vi "Initialize Source.vi"(0 "Intrument Handle[]":refnum<k15>[](array[refnum]), 2 "Channel Number":string[](array[string]), 5 "Measurement Configuration":T1={"Quick Power Down"=FALSE, "Pin Name"=[], "Source Mode"=[], "Start Value"=[], "Target Value"=[], "Compliance Limit"=[], "Sense Mode"=[], "Default Ramp Rate"=[], "Ramp Rate"=[], "Start Delay"=[], "Relative To"=[], "Transient Response"=[], "Data Capture"=FALSE, "Power line frequency"=1} {"Power line frequency" items=["50 Hz", "60 Hz"]; "Start Value" format="%#_6p"; "Transient Response" items=["Slow", "Normal", "Fast"]; "Sense Mode" items=["Local Sense", "Remote Sense"]; "Relative To" items=["Power sequence start", "Previous source start", "Previous source end"]; "Target Value" format="%#_6p"; "Source Mode" items=["DC Voltage", "DC Current"]; "Start Delay" format="%#_6p"; "Compliance Limit" format="%#_6p"; "Ramp Rate" format="%#_6p"}, 11 "error in (no error)":errorcluster) -> (4 "Intrument Handle out[]":refnum<k15>[](array[refnum]), 6 "Error":string[](array[string]), 15 "error out":errorcluster)   [LabVIEW 2024, in "devicePowerSequencerCoreLogic.lvlib"]
uses:
  devicePowerSequencerCoreLogic.lvlib
  Measurement Configuration.ctl
  controls/Source Mode.ctl
  controls/Sense Mode.ctl
  controls/Relative To.ctl
  controls/Transient Response.ctl
  controls/Power line frequency.ctl
  <instrlib>/niDCPower/nidcpower.llb/niDCPower Source Mode.ctl
  <instrlib>/niDCPower/nidcpower.llb/niDCPower Output Function.ctl
  <instrlib>/niDCPower/nidcpower.llb/niDCPower Sequence Attribute Type.ctl
  <vilib>/Utility/error.llb/Trim Whitespace.vi
  Form Error Message.vi
  <vilib>/Utility/error.llb/Trim Whitespace One-Sided.vi
  Form Error Message.vi/4da3fa3f-d6a2-4c6b-9c9c-fc44bca91f7b.vi
  <instrlib>/niDCPower/nidcpower.llb/niDCPower Create Advanced Sequence Step With Channels.vi
  <vilib>/Utility/error.llb/Error Cluster From Error Code.vi
  Device Power Sequencer.lvlib
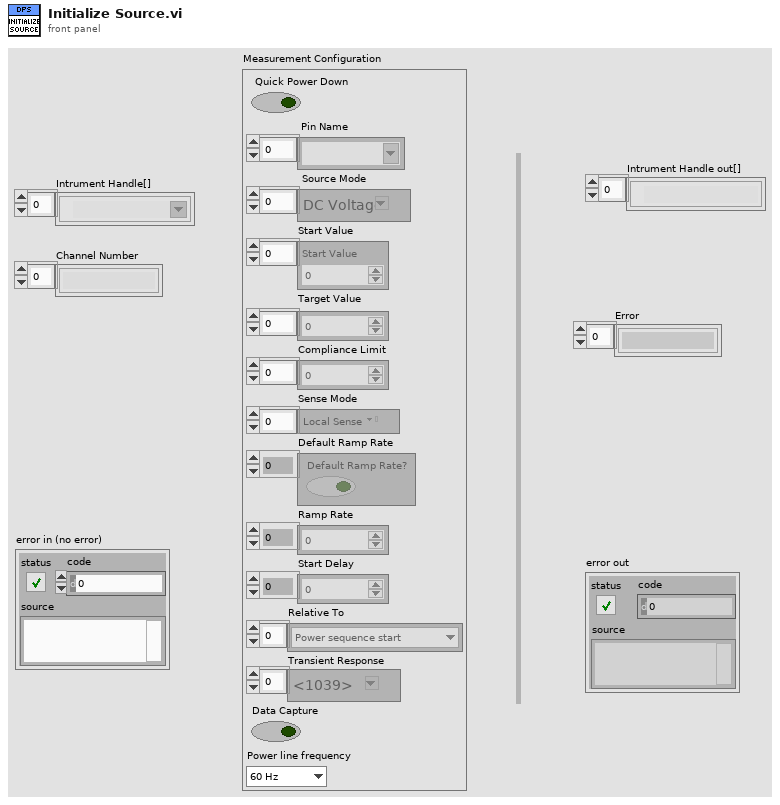
[diagram p1: front panel]
types:
  T1 = typedef "Device Power Sequencer.lvlib/Measurement Configuration.ctl" = cluster{"Quick Power Down":bool, "Pin Name":string[], "Source Mode":T2[], "Start Value":dbl[], "Target Value":dbl[], "Compliance Limit":dbl[], "Sense Mode":T3[], "Default Ramp Rate":bool[], "Ramp Rate":dbl[], "Start Delay":dbl[], "Relative To":T4[], "Transient Response":T5[], "Data Capture":bool, "Power line frequency":T6}
  T2 = typedef "Device Power Sequencer.lvlib/Source Mode.ctl" = i32
  T3 = typedef "Device Power Sequencer.lvlib/Sense Mode.ctl" = i32
  T4 = typedef "Device Power Sequencer.lvlib/Relative To.ctl" = u32
  T5 = typedef "Device Power Sequencer.lvlib/Transient Response.ctl" = i32
  T6 = typedef "Device Power Sequencer.lvlib/Power line frequency.ctl" = u32
  T7 = typedef "niDCPower Source Mode.ctl" = i32
  T8 = typedef "niDCPower Sequence Attribute Type.ctl" = i32
  T9 = typedef "niDCPower Output Function.ctl" = i32
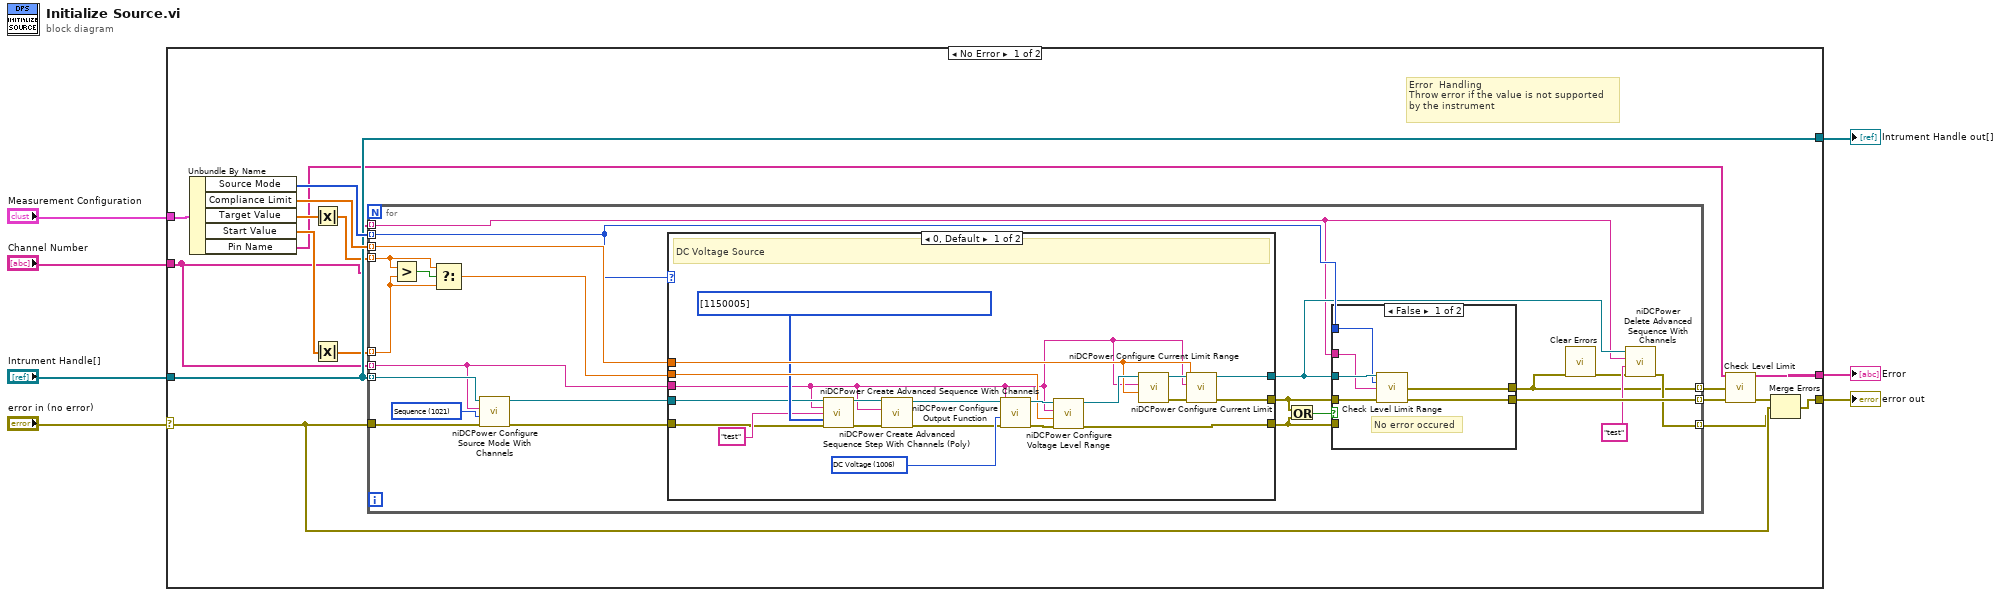
[diagram p0: block diagram]
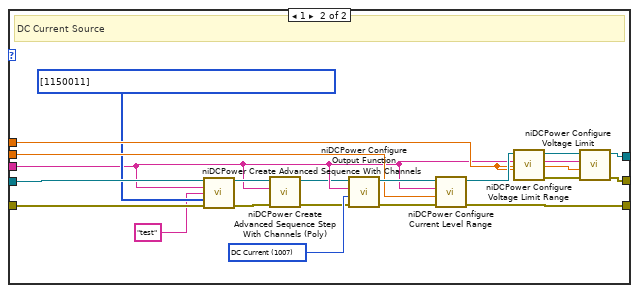
[diagram p3: hidden frame]
diagram:
  n1 = case shown="No Error" "error in (no error)" {
    selector: "error in (no error)" -> [w10 w96]
    tunnel: "Measurement Configuration" -> [w24 _]
    tunnel: "Intrument Handle[]" -> [w21 w95]
    tunnel: [w11 w96] -> w4
    tunnel: "Channel Number" -> [w9 _]
    tunnel: [w21 w95] -> w2
    tunnel: [w18 _] -> w1
    frame No Error {
      # "Error  Handling\nThrow error if the value is not supported \nby the instrument"
      n2 = Unbundle By Name(w24) -> ("Source Mode"=w23:T2[], "Compliance Limit"=w22:dbl[], "Target Value"=w17:dbl[], "Start Value"=w16:dbl[], "Pin Name"=w12:string[])
      n3 = Absolute Value(x=w17) -> (abs(x)=w19:dbl[])
      n4 = Absolute Value(x=w16) -> (abs(x)=w15:dbl[])
      n5 = for {
        tunnel: w23 -> [w41] mode=indexing
        tunnel: w21 -> [w45] mode=indexing
        tunnel: w10 -> [w44]
        tunnel: w22 -> [w43] mode=indexing
        tunnel: w9 -> [w31] mode=indexing
        tunnel: w19 -> [w36] mode=indexing
        tunnel: [w42] -> w13 mode=indexing
        tunnel: [w26] -> w14 mode=indexing
        tunnel: w15 -> [w35] mode=indexing
        tunnel: w9 -> [w29] mode=indexing
        tunnel: [w27] -> w8 mode=indexing
        w46 = T7 1021 items=["Single Point"=1020, "Sequence"=1021] ("source mode")
        n6 = Greater?(x=w36, y=w35) -> (0:w37:bool)
        n7 = Select(t=w36, s=w37, f=w35) -> (s? t:f=w34:dbl)
        n8 = call <instrlib>:"niDCPower Configure Source Mode With Channels.vi"("error in (no error)"=w44, "source mode"=w46, "channel name"=w31, "instrument handle"=w45) -> ("error out"=w33:errorcluster, "instrument handle out"=w32:refnum<k15>)  [unwired: 6 in]
        n9 = case shown="0, Default" w41 {
          tunnel: w32 -> [w60 w80]
          tunnel: w33 -> [w58 w81]
          tunnel: w43 -> [w64 w89]
          tunnel: [w69 w88] -> w39
          tunnel: w31 -> [w55 w77]
          tunnel: [w68 w85] -> w30
          tunnel: w34 -> [w67 w87]
          tunnel: [w65 w84] -> w38
          frame 0, Default {
            w63 = T8[] [1150005] items=["Source -> Output Function"=1150008, "Source -> Output Enabled"=1250006, "Source -> Output Resistance"=1150061, "Source -> Transient Response"=1150062, "Source -> Custom Transient Response -> Voltage Gain Bandwidth"=1150067, "Source -> Custom Transient Response -> Voltage Compensation Frequency"=1150068, "Source -> Custom Transient Response -> Voltage Pole-Zero Ratio"=1150069, "Source -> Custom Transient Response -> Current Gain Bandwidth"=1150070, "Source -> Custom Transient Response -> Current Compensation Frequency"=1150071, "Source -> Custom Transient Response -> Current Pole-Zero Ratio"=1150072, "Source -> DC Voltage -> Voltage Level"=1250001, "Source -> DC Voltage -> Voltage Level Range"=1150005, "Source -> DC Voltage -> Current Limit"=1250005, "Source -> DC Voltage -> Current Limit High"=1150187, "Source -> DC Voltage -> Current Limit Low"=1150188, "Source -> DC Voltage -> Current Limit Range"=1150004, "Source -> DC Current -> Current Level"=1150009, "Source -> DC Current -> Current Level Range"=1150011, "Source -> DC Current -> Voltage Limit"=1150010, "Source -> DC Current -> Voltage Limit High"=1150185, "Source -> DC Current -> Voltage Limit Low"=1150186, "Source -> DC Current -> Voltage Limit Range"=1150012, "Source -> Pulse Voltage -> Pulse Voltage Level"=1150080, "Source -> Pulse Voltage -> Pulse Bias Voltage Level"=1150082, "Source -> Pulse Voltage -> Pulse Voltage Level Range"=1150084, "Source -> Pulse Voltage -> Pulse Current Limit"=1150081, "Source -> Pulse Voltage -> Pulse Current Limit High"=1150193, "Source -> Pulse Voltage -> Pulse Current Limit Low"=1150194, "Source -> Pulse Voltage -> Pulse Bias Current Limit"=1150083, "Source -> Pulse Voltage -> Pulse Bias Current Limit High"=1150195, "Source -> Pulse Voltage -> Pulse Bias Current Limit Low"=1150196, "Source -> Pulse Voltage -> Pulse Current Limit Range"=1150085, "Source -> Pulse Current -> Pulse Current Level"=1150086, "Source -> Pulse Current -> Pulse Bias Current Level"=1150088, "Source -> Pulse Current -> Pulse Current Level Range"=1150090, "Source -> Pulse Current -> Pulse Voltage Limit"=1150087, "Source -> Pulse Current -> Pulse Voltage Limit High"=1150189, "Source -> Pulse Current -> Pulse Voltage Limit Low"=1150190, "Source -> Pulse Current -> Pulse Bias Voltage Limit"=1150089, "Source -> Pulse Current -> Pulse Bias Voltage Limit High"=1150191, "Source -> Pulse Current -> Pulse Bias Voltage Limit Low"=1150192, "Source -> Pulse Current -> Pulse Voltage Limit Range"=1150091, "Source -> Advanced -> Source Delay"=1150051, "Source -> Advanced -> Pulse Bias Delay"=1150092, "Source -> Advanced -> Pulse On Time"=1150093, "Source -> Advanced -> Pulse Off Time"=1150094, "Source -> Advanced -> OVP Enabled"=1250002, "Source -> Advanced -> OVP Limit"=1250003, "Source -> Advanced -> Compliance Limit Symmetry"=1150184, "Source -> Advanced -> Sequence Step Delta Time"=1150198, "Measurement -> Sense"=1150013, "Measurement -> Aperture Time"=1150058, "Measurement -> Measure Record Length"=1150063, "Measurement -> Advanced -> DC Noise Rejection"=1150066, "Measurement -> Autorange"=1150244, "Measurement -> Advanced -> Autorange Behavior"=1150245, "Measurement -> Advanced -> Autorange Aperture Time Mode"=1150246, "Measurement -> Advanced -> Autorange Minimum Aperture Time"=1150247, "Measurement -> Advanced -> Autorange Minimum Aperture Time Units"=1150248, "Measurement -> Advanced -> Autorange Minimum Current Range"=1150255, "Measurement -> Advanced -> Autorange Minimum Voltage Range"=1150256, "Measurement -> Advanced -> Autorange Threshold Mode"=1150257, "Measurement -> Advanced -> Autorange Maximum Delay After Range Change"=1150322, "LCR -> Instrument Mode"=1150208, "LCR -> Source Delay Mode"=1150315, "LCR -> Measurement Time"=1150218, "LCR -> Custom Measurement Time"=1150258, "LCR -> AC Stimulus -> Function"=1150209, "LCR -> AC Stimulus -> Frequency"=1150210, "LCR -> AC Stimulus -> Voltage Amplitude"=1150211, "LCR -> AC Stimulus -> Current Amplitude"=1150212, "LCR -> AC Stimulus -> Advanced -> Voltage Range"=1150265, "LCR -> AC Stimulus -> Advanced -> Current Range"=1150267, "LCR -> AC Stimulus -> Advanced -> Source Aperture Time"=1150349, "LCR -> DC Bias -> Source"=1150213, "LCR -> DC Bias -> Voltage Level"=1150214, "LCR -> DC Bias -> Current Level"=1150215, "LCR -> DC Bias -> Advanced -> Voltage Range"=1150266, "LCR -> DC Bias -> Advanced -> Current Range"=1150274, "LCR -> DC Bias -> Advanced -> Transient Response"=1150347, "LCR -> Compensation -> Open -> Enabled"=1150220, "LCR -> Compensation -> Open -> Conductance"=1150261, "LCR -> Compensation -> Open -> Susceptance"=1150262, "LCR -> Compensation -> Short -> Enabled"=1150221, "LCR -> Compensation -> Short -> Resistance"=1150263, "LCR -> Compensation -> Short -> Reactance"=1150264, "LCR -> Compensation -> Load -> Enabled"=1150222, "LCR -> Compensation -> Load -> Measured Resistance"=1150268, "LCR -> Compensation -> Load -> Measured Reactance"=1150269, "LCR -> Compensation -> Load -> Actual Resistance"=1150270, "LCR -> Compensation -> Load -> Actual Reactance"=1150271, "LCR -> Impedance Range -> Impedance Range"=1150217, "LCR -> Impedance Range -> Impedance Autorange"=1150216, "LCR -> Impedance Range -> Advanced -> Impedance Range Source"=1150321, "LCR -> Impedance Range -> Advanced -> Load Resistance"=1150318, "LCR -> Impedance Range -> Advanced -> Load Inductance"=1150319, "LCR -> Impedance Range -> Advanced -> Load Capacitance"=1150320] ("advanced sequence properties")
            w74 = T9 1006 items=["DC Voltage"=1006, "DC Current"=1007, "Pulse Voltage"=1049, "Pulse Current"=1050] ("output function")
            # "DC Voltage Source"
            n10 = call <instrlib>:"niDCPower Create Advanced Sequence With Channels.vi"("instrument handle"=w60, "channel name"=w55, "sequence name"="test", "advanced sequence properties"=w63, "error in (no error)"=w58) -> ("instrument handle out"=w62:refnum<k15>, "error out"=w61:errorcluster)  [unwired: 9 in]
            n11 = call-poly <instrlib>:"niDCPower Create Advanced Sequence Step With Channels (Poly).vi"("error in (no error)"=w61, "channel name"=w55, "instrument handle"=w62) -> ("error out"=w57:errorcluster, "instrument handle out"=w56:refnum<k15>)  [unwired: 7 in]
            n12 = call <instrlib>:"niDCPower Configure Output Function.vi"("error in (no error)"=w57, "output function"=w74, "channel name"=w55, "instrument handle"=w56) -> ("error out"=w71:errorcluster, "instrument handle out"=w73:refnum<k15>)  [unwired: 6 in]
            n13 = call <instrlib>:"niDCPower Configure Voltage Level Range.vi"("error in (no error)"=w71, "voltage level range"=w67, "channel name"=w55, "instrument handle"=w73) -> ("error out"=w65:errorcluster, "instrument handle out"=w72:refnum<k15>)  [unwired: 6 in]
            n14 = call <instrlib>:"niDCPower Configure Current Limit Range.vi"("current limit range"=w64, "channel name"=w55, "instrument handle"=w72) -> ("error out"=w66:errorcluster, "instrument handle out"=w70:refnum<k15>)  [unwired: 7 in]
            n15 = call <instrlib>:"niDCPower Configure Current Limit.vi"("error in (no error)"=w66, "current limit"=w64, "channel name"=w55, "instrument handle"=w70) -> ("error out"=w69:errorcluster, "instrument handle out"=w68:refnum<k15>)  [unwired: 6 in]
          }
          frame 1 {
            w79 = T8[] [1150011] items=["Source -> Output Function"=1150008, "Source -> Output Enabled"=1250006, "Source -> Output Resistance"=1150061, "Source -> Transient Response"=1150062, "Source -> Custom Transient Response -> Voltage Gain Bandwidth"=1150067, "Source -> Custom Transient Response -> Voltage Compensation Frequency"=1150068, "Source -> Custom Transient Response -> Voltage Pole-Zero Ratio"=1150069, "Source -> Custom Transient Response -> Current Gain Bandwidth"=1150070, "Source -> Custom Transient Response -> Current Compensation Frequency"=1150071, "Source -> Custom Transient Response -> Current Pole-Zero Ratio"=1150072, "Source -> DC Voltage -> Voltage Level"=1250001, "Source -> DC Voltage -> Voltage Level Range"=1150005, "Source -> DC Voltage -> Current Limit"=1250005, "Source -> DC Voltage -> Current Limit High"=1150187, "Source -> DC Voltage -> Current Limit Low"=1150188, "Source -> DC Voltage -> Current Limit Range"=1150004, "Source -> DC Current -> Current Level"=1150009, "Source -> DC Current -> Current Level Range"=1150011, "Source -> DC Current -> Voltage Limit"=1150010, "Source -> DC Current -> Voltage Limit High"=1150185, "Source -> DC Current -> Voltage Limit Low"=1150186, "Source -> DC Current -> Voltage Limit Range"=1150012, "Source -> Pulse Voltage -> Pulse Voltage Level"=1150080, "Source -> Pulse Voltage -> Pulse Bias Voltage Level"=1150082, "Source -> Pulse Voltage -> Pulse Voltage Level Range"=1150084, "Source -> Pulse Voltage -> Pulse Current Limit"=1150081, "Source -> Pulse Voltage -> Pulse Current Limit High"=1150193, "Source -> Pulse Voltage -> Pulse Current Limit Low"=1150194, "Source -> Pulse Voltage -> Pulse Bias Current Limit"=1150083, "Source -> Pulse Voltage -> Pulse Bias Current Limit High"=1150195, "Source -> Pulse Voltage -> Pulse Bias Current Limit Low"=1150196, "Source -> Pulse Voltage -> Pulse Current Limit Range"=1150085, "Source -> Pulse Current -> Pulse Current Level"=1150086, "Source -> Pulse Current -> Pulse Bias Current Level"=1150088, "Source -> Pulse Current -> Pulse Current Level Range"=1150090, "Source -> Pulse Current -> Pulse Voltage Limit"=1150087, "Source -> Pulse Current -> Pulse Voltage Limit High"=1150189, "Source -> Pulse Current -> Pulse Voltage Limit Low"=1150190, "Source -> Pulse Current -> Pulse Bias Voltage Limit"=1150089, "Source -> Pulse Current -> Pulse Bias Voltage Limit High"=1150191, "Source -> Pulse Current -> Pulse Bias Voltage Limit Low"=1150192, "Source -> Pulse Current -> Pulse Voltage Limit Range"=1150091, "Source -> Advanced -> Source Delay"=1150051, "Source -> Advanced -> Pulse Bias Delay"=1150092, "Source -> Advanced -> Pulse On Time"=1150093, "Source -> Advanced -> Pulse Off Time"=1150094, "Source -> Advanced -> OVP Enabled"=1250002, "Source -> Advanced -> OVP Limit"=1250003, "Source -> Advanced -> Compliance Limit Symmetry"=1150184, "Source -> Advanced -> Sequence Step Delta Time"=1150198, "Measurement -> Sense"=1150013, "Measurement -> Aperture Time"=1150058, "Measurement -> Measure Record Length"=1150063, "Measurement -> Advanced -> DC Noise Rejection"=1150066, "Measurement -> Autorange"=1150244, "Measurement -> Advanced -> Autorange Behavior"=1150245, "Measurement -> Advanced -> Autorange Aperture Time Mode"=1150246, "Measurement -> Advanced -> Autorange Minimum Aperture Time"=1150247, "Measurement -> Advanced -> Autorange Minimum Aperture Time Units"=1150248, "Measurement -> Advanced -> Autorange Minimum Current Range"=1150255, "Measurement -> Advanced -> Autorange Minimum Voltage Range"=1150256, "Measurement -> Advanced -> Autorange Threshold Mode"=1150257, "Measurement -> Advanced -> Autorange Maximum Delay After Range Change"=1150322, "LCR -> Instrument Mode"=1150208, "LCR -> Source Delay Mode"=1150315, "LCR -> Measurement Time"=1150218, "LCR -> Custom Measurement Time"=1150258, "LCR -> AC Stimulus -> Function"=1150209, "LCR -> AC Stimulus -> Frequency"=1150210, "LCR -> AC Stimulus -> Voltage Amplitude"=1150211, "LCR -> AC Stimulus -> Current Amplitude"=1150212, "LCR -> AC Stimulus -> Advanced -> Voltage Range"=1150265, "LCR -> AC Stimulus -> Advanced -> Current Range"=1150267, "LCR -> AC Stimulus -> Advanced -> Source Aperture Time"=1150349, "LCR -> DC Bias -> Source"=1150213, "LCR -> DC Bias -> Voltage Level"=1150214, "LCR -> DC Bias -> Current Level"=1150215, "LCR -> DC Bias -> Advanced -> Voltage Range"=1150266, "LCR -> DC Bias -> Advanced -> Current Range"=1150274, "LCR -> DC Bias -> Advanced -> Transient Response"=1150347, "LCR -> Compensation -> Open -> Enabled"=1150220, "LCR -> Compensation -> Open -> Conductance"=1150261, "LCR -> Compensation -> Open -> Susceptance"=1150262, "LCR -> Compensation -> Short -> Enabled"=1150221, "LCR -> Compensation -> Short -> Resistance"=1150263, "LCR -> Compensation -> Short -> Reactance"=1150264, "LCR -> Compensation -> Load -> Enabled"=1150222, "LCR -> Compensation -> Load -> Measured Resistance"=1150268, "LCR -> Compensation -> Load -> Measured Reactance"=1150269, "LCR -> Compensation -> Load -> Actual Resistance"=1150270, "LCR -> Compensation -> Load -> Actual Reactance"=1150271, "LCR -> Impedance Range -> Impedance Range"=1150217, "LCR -> Impedance Range -> Impedance Autorange"=1150216, "LCR -> Impedance Range -> Advanced -> Impedance Range Source"=1150321, "LCR -> Impedance Range -> Advanced -> Load Resistance"=1150318, "LCR -> Impedance Range -> Advanced -> Load Inductance"=1150319, "LCR -> Impedance Range -> Advanced -> Load Capacitance"=1150320] ("Array")
            w94 = T9 1007 items=["DC Voltage"=1006, "DC Current"=1007, "Pulse Voltage"=1049, "Pulse Current"=1050] ("output function")
            # "DC Current Source"
            n16 = call <instrlib>:"niDCPower Create Advanced Sequence With Channels.vi"("instrument handle"=w80, "channel name"=w77, "sequence name"="test", "advanced sequence properties"=w79, "error in (no error)"=w81) -> ("instrument handle out"=w82:refnum<k15>, "error out"=w83:errorcluster)  [unwired: 9 in]
            n17 = call-poly <instrlib>:"niDCPower Create Advanced Sequence Step With Channels (Poly).vi"("error in (no error)"=w83, "channel name"=w77, "instrument handle"=w82) -> ("error out"=w75:errorcluster, "instrument handle out"=w76:refnum<k15>)  [unwired: 7 in]
            n18 = call <instrlib>:"niDCPower Configure Output Function.vi"("error in (no error)"=w75, "output function"=w94, "channel name"=w77, "instrument handle"=w76) -> ("error out"=w93:errorcluster, "instrument handle out"=w92:refnum<k15>)  [unwired: 6 in]
            n19 = call <instrlib>:"niDCPower Configure Current Level Range.vi"("error in (no error)"=w93, "current level range"=w87, "channel name"=w77, "instrument handle"=w92) -> ("error out"=w84:errorcluster, "instrument handle out"=w90:refnum<k15>)  [unwired: 6 in]
            n20 = call <instrlib>:"niDCPower Configure Voltage Limit Range.vi"("voltage limit range"=w89, "channel name"=w77, "instrument handle"=w90) -> ("error out"=w86:errorcluster, "instrument handle out"=w91:refnum<k15>)  [unwired: 7 in]
            n21 = call <instrlib>:"niDCPower Configure Voltage Limit.vi"("error in (no error)"=w86, "voltage limit"=w89, "channel name"=w77, "instrument handle"=w91) -> ("error out"=w88:errorcluster, "instrument handle out"=w85:refnum<k15>)  [unwired: 6 in]
          }
        }
        n22 = Or(x=w39, y=w38) -> (x .or. y?=w40:bool)
        n23 = case shown="False" w40 {
          tunnel: w30 -> [w52 _]
          tunnel: w39 -> [w51 w54]
          tunnel: [w50 w53] -> w42
          tunnel: w41 -> [w49 _]
          tunnel: [w48 w54] -> w26
          tunnel: w38 -> [_ w53]
          tunnel: w29 -> [w47 _]
          frame False {
            # "No error occured"
            n24 = call "Check Level Limit Range.vi"("Intrument Handle[]"=w52, "Source Mode"=w49, "Channel Name"=w47, "error in (no error)"=w51) -> ("Error from limit"=w48:errorcluster, "Error from level"=w50:errorcluster)  [unwired: 10 in]
          }
          frame True {
            # "Error occured"
          }
        }
        n25 = call <vilib>:"Clear Errors.vi"("error in (no error)"=w26) -> ("error out"=w25:errorcluster)  [unwired: 5 in, 1 out]
        n26 = call <instrlib>:"niDCPower Delete Advanced Sequence With Channels.vi"("error in (no error)"=w25, "sequence name"="test", "channel name"=w29, "instrument handle"=w30) -> ("error out"=w27:errorcluster)  [unwired: 6 in, 1 out]
      }
      n27 = call "Check Level Limit.vi"("Pin Names"=w12, "Error from Limit"=w14, "Error from Level"=w13) -> ("Error"=w18:string[], "error out"=w20:errorcluster)  [unwired: 11 in]
      n28 = Merge Errors(w20, w10, w8) -> (w11:errorcluster)
    }
    frame Error {
    }
  }
  "error out" <- w4
  "Intrument Handle out[]" <- w2
  "Error" <- w1
